vi "(SubVI) Get Frames From Files.vi"(8 "Glimpse String Path Array":string[](array[string]), 9 "pixel# of a image":u32, 11 "pixel depth (byte)":i32) -> (3 "Frames Array":dbl[](array[numeric]))   [LabVIEW 2014]
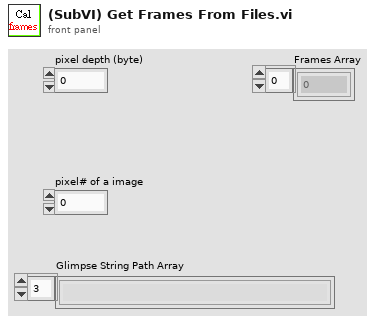
[diagram p1: front panel]
types:
  T1 = enum16{"open", "replace", "create", "open or create", "replace or create", "replace or create with confirmation"}
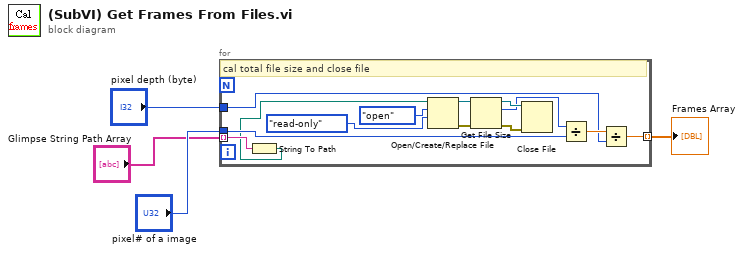
[diagram p0: block diagram]
diagram:
  n1 = for {
    tunnel: "pixel# of a image" -> [w14]
    tunnel: [w11] -> w3 mode=indexing
    tunnel: "pixel depth (byte)" -> [w12]
    tunnel: "Glimpse String Path Array" -> [w6] mode=indexing
    # "cal total file size and close file"
    n2 = String To Path(string=w6) -> (path=w5:path)
    n3 = Open/Create/Replace File(file path (use dialog)=w5, operation (0:open)=T1."open", access (0:read/write)=enum16{"read/write", "read-only", "write-only"}."read-only") -> (refnum out=w8:refnum<file>, error out=w7:errorcluster)  [unwired: 3 in, 1 out]
    n4 = Get File Size(file=w8, error in=w7) -> (refnum out=w17:refnum<file>, size (in bytes)=w15:i64, 0:w16:errorcluster)
    n5 = Close File(refnum=w17, error in=w16) -> ()  [unwired: 2 out]
    n6 = Divide(x=w15, y=w14) -> (x/y=w13:dbl)
    n7 = Divide(x=w13, y=w12) -> (x/y=w11:dbl)
  }
  "Frames Array" <- w3
